vi "EncoderTestingDriveDistance.vi"(11 "Distance":dbl) -> ()   [LabVIEW 2015]
uses:
  <vilib>/Rock Robotics/Network Tables/NT Read Number.vi
  <vilib>/addons/control/pid/pid.llb/PID (DBL).vi
  <vilib>/addons/control/pid/NI_PID_pid.lvlib
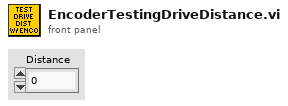
[diagram p1: front panel]
types:
  T1 = cluster{"proportional gain (Kc)":dbl, "integral time (Ti, min)":dbl, "derivative time (Td, min)":dbl}
  T2 = typedef "WPI_EncoderDevRef.ctl" = cluster{"DevStatus":errorcluster, "EncoderIndex":T3, "CounterIndex":T4, "DistancePerCount":dbl, "Decoding Type":T5}
  T3 = typedef "FPGA_EncoderIdx.ctl" = enum8{"Enc 0", "Enc 1", "Enc 2", "Enc 3", "Enc 4", "Enc 5", "Enc 6", "Enc 7", "Invalid"}
  T4 = typedef "FPGA_CounterCtrSystemIndex.ctl" = enum8{"Ctr 0", "Ctr 1", "Ctr 2", "Ctr 3", "Ctr 4", "Ctr 5", "Ctr 6", "Ctr 7", "Invalid"}
  T5 = typedef "WPI_EncoderType.ctl" = enum16{"1x", "2x", "4x"}
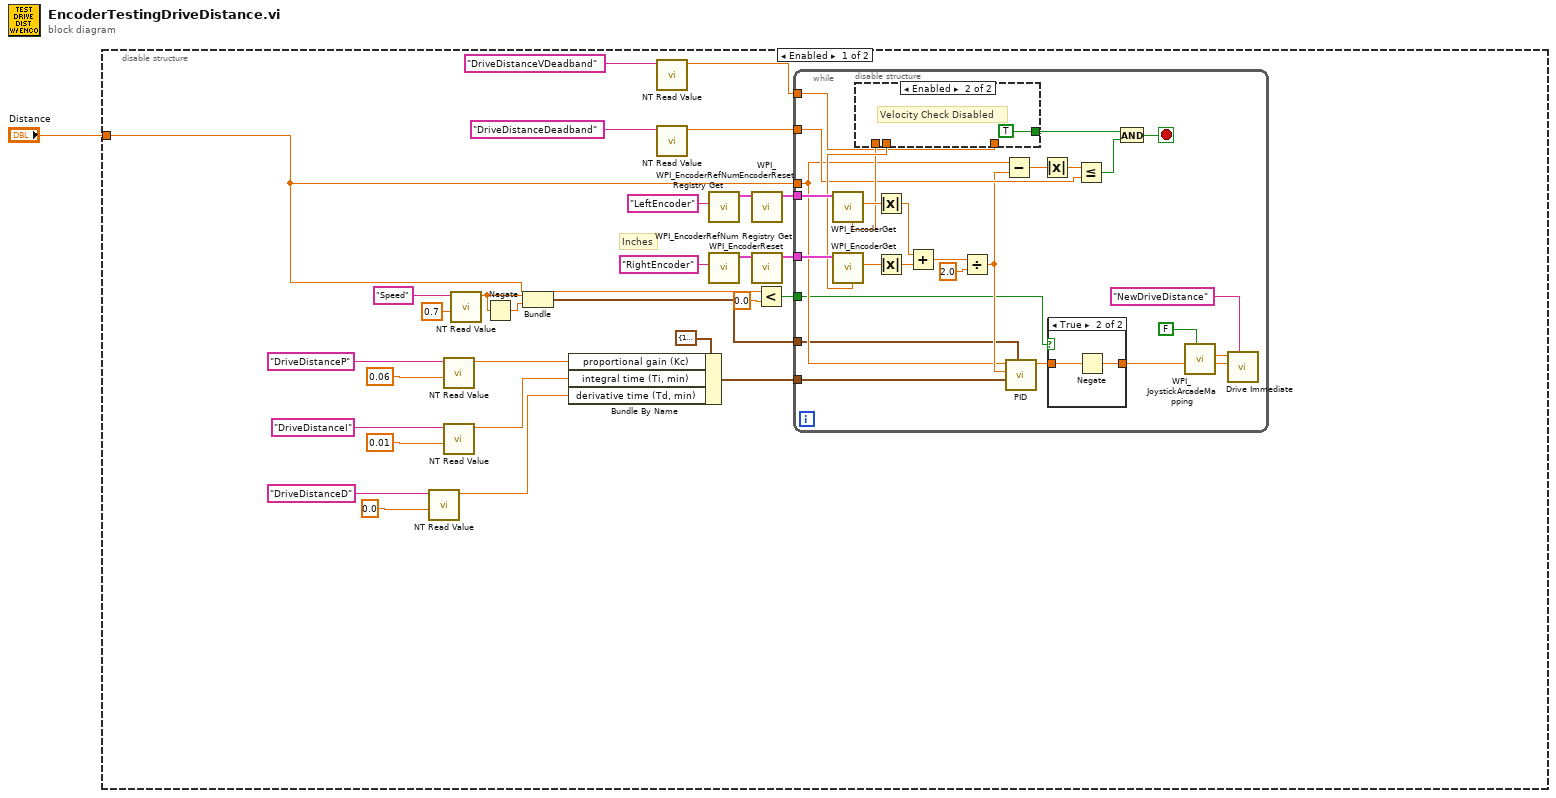
[diagram p0: block diagram]
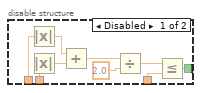
[diagram p2: hidden frame]
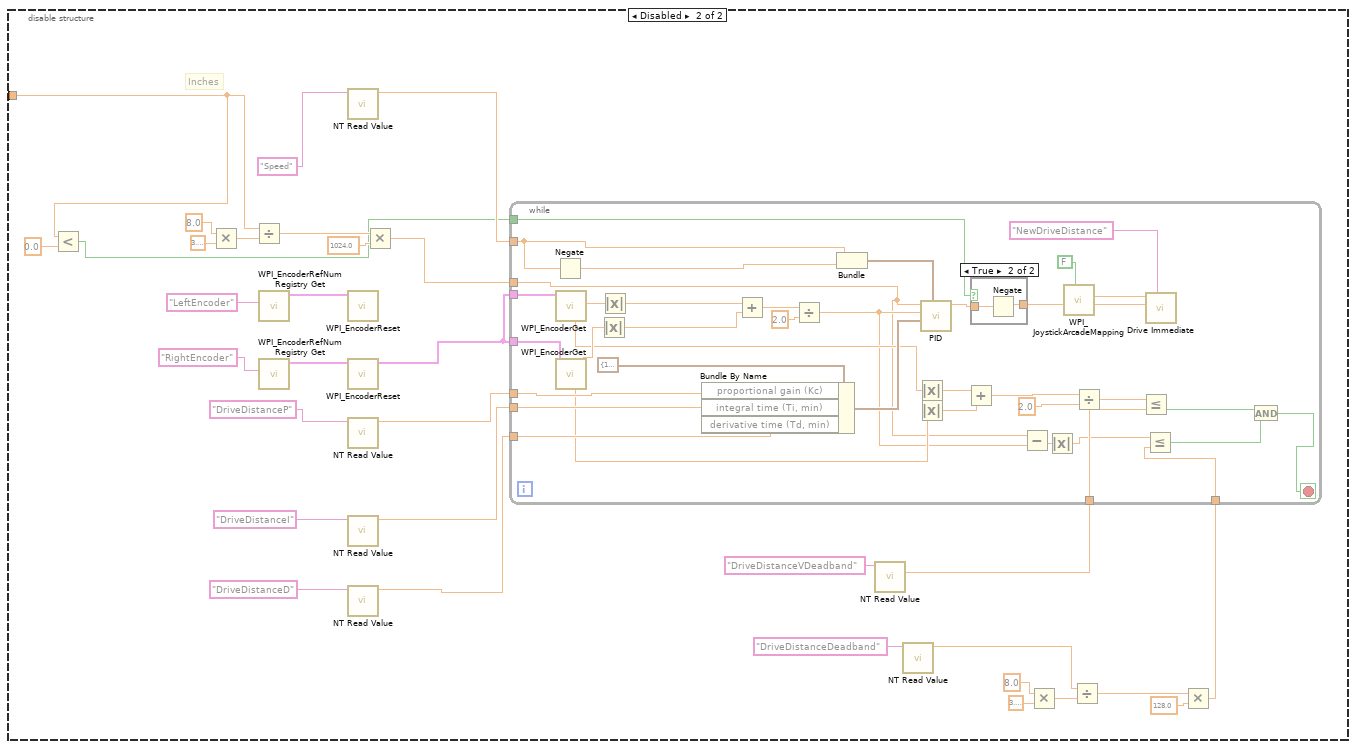
[diagram p4: hidden frame]
diagram:
  n1 = disable-structure shown="Enabled" {
    disable-tunnel: "Distance" -> [w17 w74]
    frame Enabled {
      # "Inches"
      n2 = call-poly <vilib>:"NT Read Value.vi"("Default Value"=0.0, "Name"="DriveDistanceD") -> ("Numeric"=w5:dbl)  [unwired: 8 in, 1 out]
      n3 = call-poly <vilib>:"NT Read Value.vi"("Default Value"=0.06, "Name"="DriveDistanceP") -> ("Numeric"=w7:dbl)  [unwired: 8 in, 1 out]
      n4 = call-poly <vilib>:"NT Read Value.vi"("Default Value"=0.01, "Name"="DriveDistanceI") -> ("Numeric"=w6:dbl)  [unwired: 8 in, 1 out]
      n5 = call-poly <vilib>:"NT Read Value.vi"("Default Value"=0.7, "Name"="Speed") -> ("Numeric"=w9:dbl)  [unwired: 8 in, 1 out]
      n6 = Negate(x=w9) -> (-x=w10:dbl)
      n7 = Bundle("Numeric"=w9, w10) -> (w8:cluster{"Numeric":dbl, dbl})  [unwired: 1 in]
      n8 = Bundle By Name(cluster=T1 {"proportional gain (Kc)"=1.0, "integral time (Ti, min)"=0.01, "derivative time (Td, min)"=0.0} ("PID gains"), "proportional gain (Kc)"=w7, "integral time (Ti, min)"=w6, "derivative time (Td, min)"=w5) -> (w4:T1)
      n9 = call-poly <vilib>:"NT Read Value.vi"("Name"="DriveDistanceVDeadband") -> ("Numeric"=w20:dbl)  [unwired: 9 in, 1 out]
      n10 = call-poly <vilib>:"NT Read Value.vi"("Name"="DriveDistanceDeadband") -> ("Numeric"=w18:dbl)  [unwired: 9 in, 1 out]
      n11 = call <vilib>:"WPI_EncoderRefNum Registry Get.vi"("refnum name"="LeftEncoder") -> ("EncoderDevRef"=w30:T2)  [unwired: 9 in, 1 out]
      n12 = call <vilib>:"WPI_EncoderRefNum Registry Get.vi"("refnum name"="RightEncoder") -> ("EncoderDevRef"=w29:T2)  [unwired: 9 in, 1 out]
      n13 = call <vilib>:"WPI_EncoderReset.vi"("EncoderDevRef"=w30) -> ("EncoderDevRef"=w14:T2)  [unwired: 9 in, 1 out]
      n14 = call <vilib>:"WPI_EncoderReset.vi"("EncoderDevRef"=w29) -> ("EncoderDevRef"=w19:T2)  [unwired: 9 in, 1 out]
      n15 = Less?(x=w17, y=0.0) -> (x < y?=w15:bool)
      n16 = while {
        tunnel: w14 -> [w58]
        tunnel: w19 -> [w57]
        tunnel: w17 -> [w40]
        tunnel: w20 -> [w46]
        tunnel: w18 -> [w42]
        tunnel: w15 -> [w33]
        tunnel: w8 -> [w32]
        tunnel: w4 -> [w31]
        stop <- w45 stop-if-true
        n17 = call <vilib>:"WPI_EncoderGet.vi"("EncoderDevRef"=w58) -> ("Distance"=w49:dbl, "Rate"=w47:dbl)  [unwired: 5 in, 4 out]
        n18 = call <vilib>:"WPI_EncoderGet.vi"("EncoderDevRef"=w57) -> ("Distance"=w56:dbl, "Rate"=w48:dbl)  [unwired: 5 in, 4 out]
        n19 = disable-structure shown="Enabled" {
          disable-tunnel: w48 -> [w63 _]
          disable-tunnel: w47 -> [w62 _]
          disable-tunnel: w46 -> [w60 _]
          disable-tunnel: [w59 TRUE] -> w44
          frame Disabled {
            n20 = Absolute Value(x=w62) -> (abs(x)=w65:dbl)
            n21 = Absolute Value(x=w63) -> (abs(x)=w64:dbl)
            n22 = Add(x=w65, y=w64) -> (x+y=w67:dbl)
            n23 = Divide(x=w67, y=2.0) -> (x/y=w61:dbl)
            n24 = Less Or Equal?(x=w61, y=w60) -> (x <= y?=w59:bool)
          }
          frame Enabled {
            # "Velocity Check Disabled"
          }
        }
        n25 = Absolute Value(x=w49) -> (abs(x)=w37:dbl)
        n26 = Absolute Value(x=w56) -> (abs(x)=w36:dbl)
        n27 = Add(x=w37, y=w36) -> (x+y=w55:dbl)
        n28 = Divide(x=w55, y=2.0) -> (x/y=w41:dbl)
        n29 = Subtract(x=w40, y=w41) -> (x-y=w39:dbl)
        n30 = call-poly <vilib>:"PID.vi"("output range"=w32, "PID gains"=w31, "process variable"=w41, "setpoint"=w40) -> ("output"=w35:dbl)  [unwired: 6 in, 1 out]
        n31 = Absolute Value(x=w39) -> (abs(x)=w38:dbl)
        n32 = case shown="True" w33 {
          tunnel: w35 -> [w69 w70]
          tunnel: [w69 w71] -> w34
          frame False {
          }
          frame True {
            n33 = Negate(x=w70) -> (-x=w71:dbl)
          }
        }
        n34 = Less Or Equal?(x=w38, y=w42) -> (x <= y?=w43:bool)
        n35 = And(x=w44, y=w43) -> (x .and. y?=w45:bool)
        n36 = call <vilib>:"WPI_JoystickArcadeMapping.vi"("Square Inputs"=FALSE, "Y axis value"=w34) -> ("Right Motor Value"=w52:dbl, "Left Motor Value"=w51:dbl)  [unwired: 8 in]
        n37 = call "Drive Immediate.vi"("Description"="NewDriveDistance", "Right Setpoint"=w52, "Left Setpoint"=w51) -> ()  [unwired: 8 in, 1 out]
      }
    }
    frame Disabled {
      # "Inches"
      n38 = Less?(x=w74, y=0.0) -> (x < y?=w72:bool)
      n39 = Multiply(x=8.0, y=3.141592653589793) -> (x*y=w97:dbl)
      n40 = Divide(x=w74, y=w97) -> (x/y=w96:dbl)
      n41 = call <vilib>:"WPI_EncoderRefNum Registry Get.vi"("refnum name"="LeftEncoder") -> ("EncoderDevRef"=w103:T2)  [unwired: 9 in, 1 out]
      n42 = call <vilib>:"WPI_EncoderRefNum Registry Get.vi"("refnum name"="RightEncoder") -> ("EncoderDevRef"=w102:T2)  [unwired: 9 in, 1 out]
      n43 = call-poly <vilib>:"NT Read Value.vi"("Name"="Speed") -> ("Numeric"=w92:dbl)  [unwired: 9 in, 1 out]
      n44 = call <vilib>:"WPI_EncoderReset.vi"("EncoderDevRef"=w103) -> ()  [unwired: 9 in, 2 out]
      n45 = call <vilib>:"WPI_EncoderReset.vi"("EncoderDevRef"=w102) -> ("EncoderDevRef"=w82:T2)  [unwired: 9 in, 1 out]
      n46 = call-poly <vilib>:"NT Read Value.vi"("Name"="DriveDistanceP") -> ("Numeric"=w87:dbl)  [unwired: 9 in, 1 out]
      n47 = call-poly <vilib>:"NT Read Value.vi"("Name"="DriveDistanceI") -> ("Numeric"=w86:dbl)  [unwired: 9 in, 1 out]
      n48 = call-poly <vilib>:"NT Read Value.vi"("Name"="DriveDistanceD") -> ("Numeric"=w85:dbl)  [unwired: 9 in, 1 out]
      n49 = Multiply(x=w96, y=1024.0) -> (x*y=w91:dbl)
      n50 = call-poly <vilib>:"NT Read Value.vi"("Name"="DriveDistanceVDeadband") -> ("Numeric"=w83:dbl)  [unwired: 9 in, 1 out]
      n51 = call-poly <vilib>:"NT Read Value.vi"("Name"="DriveDistanceDeadband") -> ("Numeric"=w76:dbl)  [unwired: 9 in, 1 out]
      n52 = Multiply(x=8.0, y=3.141592653589793) -> (x*y=w79:dbl)
      n53 = Divide(x=w76, y=w79) -> (x/y=w78:dbl)
      n54 = Multiply(x=w78, y=128.0) -> (x*y=w75:dbl)
      n55 = while {
        tunnel: w82 -> [w142]
        tunnel: w82 -> [w141]
        tunnel: w92 -> [w136]
        tunnel: w91 -> [w111]
        tunnel: w87 -> [w133]
        tunnel: w86 -> [w132]
        tunnel: w85 -> [w131]
        tunnel: w83 -> [w117]
        tunnel: w75 -> [w113]
        tunnel: w72 -> [w104]
        stop <- w116 stop-if-true
        n56 = Negate(x=w136) -> (-x=w137:dbl)
        n57 = call <vilib>:"WPI_EncoderGet.vi"("EncoderDevRef"=w142) -> ("Distance"=w125:dbl, "Rate"=w119:dbl)  [unwired: 5 in, 4 out]
        n58 = call <vilib>:"WPI_EncoderGet.vi"("EncoderDevRef"=w141) -> ("Distance"=w140:dbl, "Rate"=w120:dbl)  [unwired: 5 in, 4 out]
        n59 = Absolute Value(x=w140) -> (abs(x)=w107:dbl)
        n60 = Absolute Value(x=w125) -> (abs(x)=w108:dbl)
        n61 = Bundle By Name(cluster=T1 {"proportional gain (Kc)"=1.0, "integral time (Ti, min)"=0.01, "derivative time (Td, min)"=0.0} ("PID gains"), "proportional gain (Kc)"=w133, "integral time (Ti, min)"=w132, "derivative time (Td, min)"=w131) -> (w130:T1)
        n62 = Add(x=w108, y=w107) -> (x+y=w139:dbl)
        n63 = Divide(x=w139, y=2.0) -> (x/y=w112:dbl)
        n64 = Bundle("Numeric"=w136, w137) -> (w135:cluster{"Numeric":dbl, dbl})  [unwired: 1 in]
        n65 = Absolute Value(x=w119) -> (abs(x)=w122:dbl)
        n66 = Absolute Value(x=w120) -> (abs(x)=w121:dbl)
        n67 = call-poly <vilib>:"PID.vi"("output range"=w135, "PID gains"=w130, "process variable"=w112, "setpoint"=w111) -> ("output"=w106:dbl)  [unwired: 6 in, 1 out]
        n68 = Add(x=w122, y=w121) -> (x+y=w124:dbl)
        n69 = case shown="True" w104 {
          tunnel: w106 -> [w143 w144]
          tunnel: [w143 w145] -> w105
          frame False {
          }
          frame True {
            n70 = Negate(x=w144) -> (-x=w145:dbl)
          }
        }
        n71 = Subtract(x=w111, y=w112) -> (x-y=w110:dbl)
        n72 = Absolute Value(x=w110) -> (abs(x)=w109:dbl)
        n73 = call <vilib>:"WPI_JoystickArcadeMapping.vi"("Square Inputs"=FALSE, "Y axis value"=w105) -> ("Right Motor Value"=w128:dbl, "Left Motor Value"=w127:dbl)  [unwired: 8 in]
        n74 = Divide(x=w124, y=2.0) -> (x/y=w118:dbl)
        n75 = Less Or Equal?(x=w118, y=w117) -> (x <= y?=w115:bool)
        n76 = Less Or Equal?(x=w109, y=w113) -> (x <= y?=w114:bool)
        n77 = call "Drive Immediate.vi"("Description"="NewDriveDistance", "Right Setpoint"=w128, "Left Setpoint"=w127) -> ()  [unwired: 8 in, 1 out]
        n78 = And(x=w115, y=w114) -> (x .and. y?=w116:bool)
      }
    }
  }
